vi "hamamatsuFrameCounterOpen.vi"   [LabVIEW 2017]
uses:
  globalDevices.vi
  <vilib>/DAQmx/create/channels.llb/DAQmx Create Channel (CI-Count Edges).vi
  <resource>/objmgr/daqmx.rc
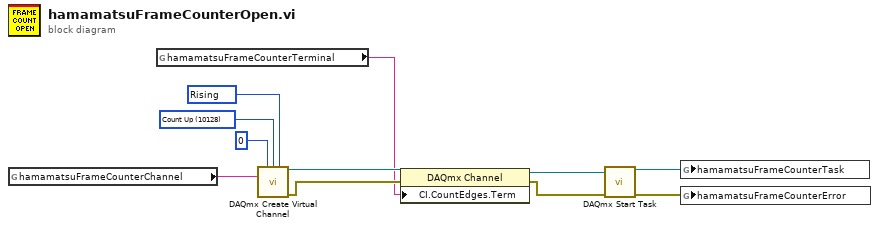
[diagram p0: block diagram]
diagram:
  w8 = 10280 items=["Rising"=10280, "Falling"=10171] ("edge")
  w9 = 10128 items=["Count Up"=10128, "Count Down"=10124, "Externally Controlled"=10326] ("count direction")
  n1 = global read "globalDevices.vi" "hamamatsuFrameCounterChannel"() -> (w11:tag)
  n2 = global read "globalDevices.vi" "hamamatsuFrameCounterTerminal"() -> (w1:tag)
  n3 = call-poly <vilib>:"DAQmx Create Virtual Channel.vi"("initial count"=u32 0, "count direction"=w9, "edge"=w8, "counter"=w11) -> ("task out"=w5:refnum<k21>, "error out"=w4:errorcluster)  [unwired: 10 in]
  n4 = property class="DAQmx Channel"(reference=w5, error in=w4, "CI.CountEdges.Term"=w1) -> (reference out=w3:refnum<k21>, error out=w2:errorcluster)
  n5 = call <vilib>:"DAQmx Start Task.vi"("task/channels in"=w3, "error in"=w2) -> ("task out"=w7:refnum<k21>, "error out"=w6:errorcluster)  [unwired: 12 in]
  n6 = global write "globalDevices.vi" "hamamatsuFrameCounterTask"(w7) -> ()
  n7 = global write "globalDevices.vi" "hamamatsuFrameCounterError"(w6) -> ()
